vi "INIT swerve.vi"(8 "error in (no error)":errorcluster) -> (0 "error out":errorcluster)   [LabVIEW 2023]
uses:
  <vilib>/Rock Robotics/WPI/ThirdParty/Phoenix-LabVIEW/Motor Controller/Controls/CTRE_Phoenix_MotorControl_ControlMode.ctl
  <vilib>/Rock Robotics/WPI/ThirdParty/REV Robotics/REVLib/Typedef/Spark MAX Control Type.ctl
  Global INIT.vi
panel:
  in  "limit SWERVE TO FIRST\nMODULE ONLY for TESTING":bool=TRUE
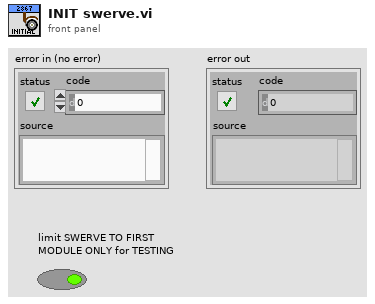
[diagram p1: front panel]
types:
  T1 = typedef "ctrl swerve motor.ctl" = cluster{"description":string, "MOTOR SELECT":T2, "Installed?":bool, "CAN ID":u8, "refnum name":string, "Invert":bool, "Idle Mode":T3, "Current limiting":T4, "MOTOR PIDF coefficients":T5, "gear ratio":dbl}
  T2 = typedef "ctrl MOTOR SELECT.ctl" = i16
  T3 = typedef "Spark MAX Idle Mode.ctl" = enum16{"Coast", "Brake"}
  T4 = typedef "ctrl Spark MAX current limiting.ctl" = cluster{"Linearized":bool, "Free Speed (A)":dbl, "Primay (A)":dbl, "Limit RPM (0)":u32}
  T5 = typedef "ctrl motor PIDF coefficients.ctl" = cluster{"PIDF":cluster{"P Gain":dbl, "I Gain":dbl, "D Gain":dbl, "F Gain":dbl, "I Zone":dbl, "Min Output":dbl, "Max Output":dbl}, "Smart Motion":T6}
  T6 = typedef "Spark MAX Smart Motion Parameters.ctl" = cluster{"Max Velocity":dbl, "Max Acceleration":dbl, "Minimum Velocity Output":dbl, "Allowed Closed Loop Error":dbl}
  T7 = typedef "ctrl Talon FX config.ctl" = cluster{"refnum name":string, "CAN ID":u8, "Installed?":bool, "description":string, "MOTOR SELECT":T2, "CAN Bus":string, "Invert Type":T8, "Neutral Mode":T9, "gear ratio":dbl, "MOTOR PIDF coefficients":T5, "Throttle":cluster{"Ramp Open (s)":dbl, "Ramp Closed (s)":dbl, "Percent Deadband":dbl}, "Supply Current Limits":cluster{"Enable?":bool, "Current Limit":dbl, "Threshold Current":dbl, "Threshold Time":dbl}}
  T8 = typedef "CTRE_Phoenix_MotorControl_TalonFXInvertType.ctl" = enum16{"Counter-Clockwise", "Clockwise"}
  T9 = typedef "CTRE_Phoenix_MotorControl_NeutralMode.ctl" = enum8{"EEPROMSetting", "Override to Coast", "Override to Brake"}
  T10 = typedef "ctrl CANcoder.ctl" = cluster{"description":string, "Installed?":bool, "CAN ID":u8, "CAN Bus":string, "refnum name":string, "Sensor Direction":bool, "Magnet Offset (Degrees)":dbl, "gear ratio":dbl}
  T11 = typedef "Spark MAX Control Type.ctl" = enum16{"Percent VBus", "Voltage", "Velocity", "Position", "Smart Motion", "Current", "Smart Velocity", "MAXMotion Position", "MAXMotion Velocity"}
  T12 = typedef "WPI_MotorControlDeviceRef.ctl" = cluster{"DeviceStatus":errorcluster, "Type":T13, "PWM":cluster{"PWM Channel":T14, "DeadBand":T15}, "CAN":cluster{"Device Number":u8, "SetOutput VI Ref":variant, "GetOutput VI Ref":variant, "Enable VI Ref":variant, "Disable VI Ref":variant, "Data":variant}, "Invert":bool, "DIO PWM":cluster{"PWM \"Enable\" Channel":T14, "DIOChannel":T16, "PWM Rate":dbl}}
  T13 = typedef "WPI_MotorControlType.ctl" = enum16{"PWM", "CAN", "DIO PWM"}
  T14 = typedef "FPGA_DIOPWMChannel.ctl" = enum8{"PWM 0", "PWM 1", "PWM 2", "PWM 3", "PWM 4", "PWM 5", "PWM 6", "PWM 7", "PWM 8", "PWM 9", "PWM MXP 0", "PWM MXP 1", "PWM MXP 2", "PWM MXP 3", "PWM MXP 4", "PWM MXP 5", "PWM MXP 6", "PWM MXP 7", "PWM MXP 8", "PWM MXP 9", "Invalid"}
  T15 = typedef "WPI_PWMDeadband.ctl" = cluster{"Name":string, "maxPositivePwm":i32, "minPositivePwm":i32, "centerPwm":i32, "maxNegativePwm":i32, "minNegativePwm":i32, "angularRange":u16}
  T16 = typedef "FPGA_DIOChannel.ctl" = enum8{"DIO 0", "DIO 1", "DIO 2", "DIO 3", "DIO 4", "DIO 5", "DIO 6", "DIO 7", "DIO 8", "DIO 9", "DIO MXP 0", "DIO MXP 1", "DIO MXP 2", "DIO MXP 3", "DIO MXP 4", "DIO MXP 5", "DIO MXP 6", "DIO MXP 7", "DIO MXP 8", "DIO MXP 9", "DIO MXP 10", "DIO MXP 11", "DIO MXP 12", "DIO MXP 13", "DIO MXP 14", "DIO MXP 15", "SPI Port CS1", "SPI Port CS2", "SPI Port CS3", "SPI Port MISO", "SPI Port MOSI", "Invalid"}
  T17 = typedef "CTRE_Phoenix_MotorControl_ControlMode.ctl" = u16
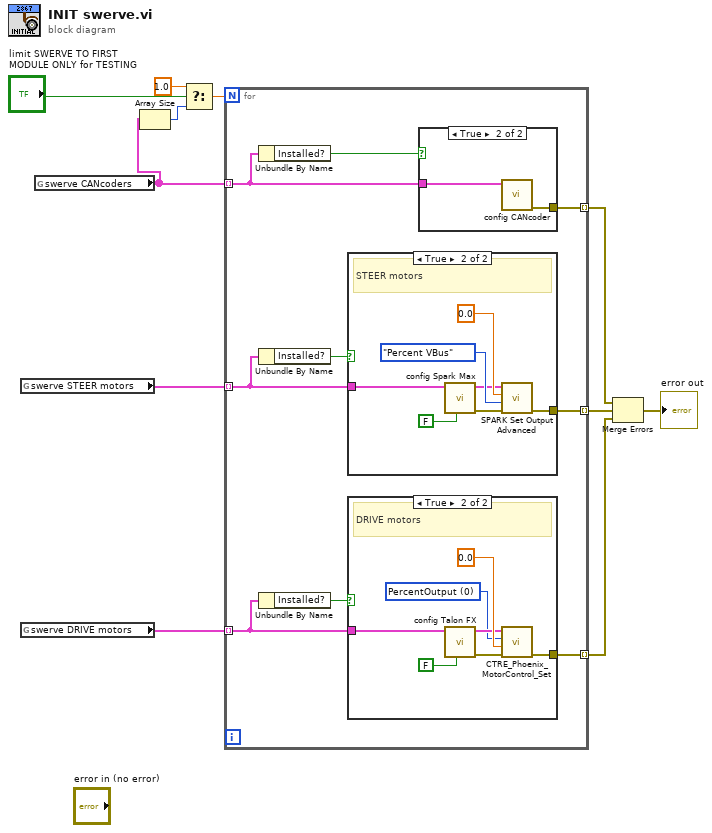
[diagram p0: block diagram]
diagram:
  n1 = global read "Global INIT.vi" "swerve STEER motors"() -> (w10:T1[])
  n2 = global read "Global INIT.vi" "swerve DRIVE motors"() -> (w11:T7[])
  n3 = global read "Global INIT.vi" "swerve CANcoders"() -> (w1:T10[])
  n4 = Array Size(array=w1) -> (size(s)=w2:i32)
  n5 = Select(t=1.0, s="limit SWERVE TO FIRST\nMODULE ONLY for TESTING", f=w2) -> (s? t:f=w5:dbl)
  n6 = for {
    N: w5 -> [_]
    tunnel: w10 -> [w18] mode=indexing
    tunnel: w1 -> [w16] mode=indexing
    tunnel: w11 -> [w19] mode=indexing
    tunnel: [w14] -> w8 mode=indexing
    tunnel: [w13] -> w7 mode=indexing
    tunnel: [w12] -> w9 mode=indexing
    n7 = Unbundle By Name(w16) -> ("Installed?"=w15:bool)
    n8 = Unbundle By Name(w18) -> ("Installed?"=w17:bool)
    n9 = Unbundle By Name(w19) -> ("Installed?"=w20:bool)
    n10 = case shown="True" w17 {
      tunnel: w18 -> [_ w27]
      tunnel: [_ w23] -> w14
      frame False {
      }
      frame True {
        # "STEER motors"
        n11 = call "config Spark Max.vi"("LIMIT SW\nEnabled?"=FALSE ("LIMIT SW\nEnabled?"), "motor\ndefaults"=w27) -> ("error out"=w24:errorcluster, "MotorControlDevRef"=w25:T12)  [unwired: 8 in]
        n12 = call <vilib>:"SPARK Set Output Advanced.vi"("error in (no error)"=w24, "Control Mode"=Spark_MAX_Control_Type."Percent VBus", "Setpoint"=0.0 ("Output"), "MotorControlDevRef"=w25) -> ("error out"=w23:errorcluster)  [unwired: 6 in, 1 out]
      }
    }
    n13 = case shown="True" w20 {
      tunnel: w19 -> [_ w35]
      tunnel: [_ w31] -> w13
      frame False {
      }
      frame True {
        w30 = T17 0 items=["PercentOutput"=0, "Position"=1, "Velocity"=2, "Current"=3, "Follower"=5, "MotionProfile"=6, "MotionMagic"=7, "MotionProfileArc"=10, "Disabled"=15] ("Control Mode")
        # "DRIVE motors"
        n14 = call "config Talon FX.vi"("LIMIT SW\nEnabled?"=FALSE ("LIMIT SW\nEnabled?"), "Talon FX motor defaults"=w35) -> ("error out"=w33:errorcluster, "PhoenixMotorControlDevRef"=w34:T12)  [unwired: 8 in]
        n15 = call <vilib>:"CTRE_Phoenix_MotorControl_Set.vi"("error in (no error)"=w33, "Output"=0.0, "Control Mode"=w30, "PhoenixMotorControlDevRef"=w34) -> ("error out"=w31:errorcluster)  [unwired: 6 in, 1 out]
      }
    }
    n16 = case shown="True" w15 {
      tunnel: w16 -> [_ w22]
      tunnel: [_ w21] -> w12
      frame False {
      }
      frame True {
        n17 = call "config CANcoder.vi"("CANcoder init data"=w22) -> ("error out"=w21:errorcluster)  [unwired: 10 in]
      }
    }
  }
  n18 = Merge Errors(w9, w8, w7) -> (→"error out":errorcluster)
